vi "test_read-nmea-data2.vi"() -> ()   [LabVIEW 2019] (continued)
\t$GPGSV,3,2,09,09,45,074,34,12,24,277,32,17,33,153,39,19,53,157,39,1*6A\n\t\n15:11:33.42\tF9P\t$GPGSV,3,3,09,25,12,307,18,1*54\n\t\n15:11:33.44\tF9P\t$GPGSV,3,1,09,02,54,318,,04,18,044,,05,37,247,,06,64,047,22,6*6B\n\t\n15:11:33.46\tF9P\t$GPGSV,3,2,09,09,45,074,24,12,24,277,,17,33,153,23,19,53,157,,6*6C\n\t\n15:11:33.48\tF9P\t$GPGSV,3,3,09,25,12,307,,6*5A\n\t\n15:11:33.50\tF9P\t$GLGSV,2,1,08,69,12,031,,70,71,039,,71,52,205,32,72,04,209,,1*7B\n\t\n15:11:33.52\tF9P\t$GLGSV,2,2,08,77,01,326,,84,20,122,13,85,70,065,34,86,36,330,,1*7E\n\t\n15:11:33.54\tF9P\t$GLGSV,2,1,08,69,12,031,,70,71,039,,71,52,205,26,72,04,209,,3*7C\n\t\n15:11:33.56\tF9P\t$GLGSV,2,2,08,77,01,326,,84,20,122,17,85,70,065,23,86,36,330,,3*7E\n\t\n15:11:33.58\tF9P\t$GAGSV,2,1,08,02,08,297,08,04,66,118,32,09,32,193,25,11,71,358,20,7*75\n\t\n15:11:33.60\tF9P\t$GAGSV,2,2,08,12,40,102,32,19,26,045,19,25,09,249,,36,26,308,23,7*71\n\t\n15:11:33.62\tF9P\t$GAGSV,2,1,08,02,08,297,,04,66,118,,09,32,193,,11,71,358,,2*7C\n\t\n15:11:33.64\tF9P\t$GAGSV,2,2,08,12,40,102,,19,26,045,,25,09,249,,36,26,308,,2*7C\n\t\n15:11:33.66\tF9P\t$GBGSV,1,1,03,11,50,132,33,14,87,127,26,33,60,219,25,1*41\n\t\n15:11:33.68\tF9P\t$GBGSV,1,1,03,11,50,132,26,14,87,127,,33,60,219,,3*44\n\t\n15:11:33.70\tF9P\t$GNGLL,3723.52856,N,12656.91091,E,061135.00,A,A*78\n\t\n15:11:33.72\tF9P\t\t\n15:11:33.74\tF9P\t\t\n15:11:33.76\tF9P\t\t\n15:11:33.78\tF9P\t\t\n15:11:33.80\tF9P\t\t\n15:11:33.84\tF9P\t\t\n15:11:33.86\tF9P\t\t\n15:11:33.88\tF9P\t\t\n15:11:33.90\tF9P\t\t\n15:11:33.92\tF9P\t\t\n15:11:33.94\tF9P\t\t\n15:11:33.96\tF9P\t\t\n15:11:33.98\tF9P\t\t\n15:11:34.00\tF9P\t\t\n15:11:34.02\tF9P\t\t\n15:11:34.04\tF9P\t\t\n15:11:34.06\tF9P\t\t\n15:11:34.08\tF9P\t\t\n15:11:34.10\tF9P\t\t\n15:11:34.12\tF9P\t\t\n15:11:34.14\tF9P\t\t\n15:11:34.16\tF9P\t\t\n15:11:34.18\tF9P\t\t\n15:11:34.20\tF9P\t\t\n15:11:34.22\tF9P\t\t\n15:11:34.24\tF9P\t$GNRMC,061136.00,A,3723.52804,N,12656.91189,E,2.935,120.29,250720,,,A,V*0E\n\t\n15:11:34.26\tF9P\t$GNVTG,120.29,T,,M,2.935,N,5.436,K,A*22\n\t\n15:11:34.28\tF9P\t$GNGGA,061136.00,3723.52804,N,12656.91189,E,1,12,0.68,33.7,M,18.5,M,,*77\n\t\n15:11:34.30\tF9P\t$GNGSA,A,3,12,06,19,05,17,09,04,02,,,,,1.27,0.68,1.08,1*03\n\t\n15:11:34.32\tF9P\t$GNGSA,A,3,85,71,84,,,,,,,,,,1.27,0.68,1.08,2*06\n\t\n15:11:34.34\tF9P\t$GNGSA,A,3,36,19,11,04,09,12,,,,,,,1.27,0.68,1.08,3*03\n\t\n15:11:34.36\tF9P\t$GNGSA,A,3,14,11,33,,,,,,,,,,1.27,0.68,1.08,4*02\n\t\n15:11:34.38\tF9P\t$GPGSV,3,1,09,02,54,318,27,04,18,044,29,05,37,247,21,06,64,047,25,1*66\n\t\n15:11:34.40\tF9P\t$GPGSV,3,2,09,09,45,074,38,12,24,277,31,17,33,153,37,19,53,157,33,1*61\n\t\n15:11:34.42\tF9P\t$GPGSV,3,3,09,25,12,307,17,1*5B\n\t\n15:11:34.44\tF9P\t$GPGSV,3,1,09,02,54,318,,04,18,044,27,05,37,247,,06,64,047,21,6*6D\n\t\n15:11:34.46\tF9P\t$GPGSV,3,2,09,09,45,074,23,12,24,277,,17,33,153,23,19,53,157,,6*6B\n\t\n15:11:34.48\tF9P\t$GPGSV,3,3,09,25,12,307,,6*5A\n\t\n15:11:34.50\tF9P\t$GLGSV,2,1,08,69,12,031,,70,71,039,,71,52,205,28,72,04,209,,1*70\n\t\n15:11:34.52\tF9P\t$GLGSV,2,2,08,77,01,326,,84,20,122,10,85,70,065,35,86,36,330,,1*7C\n\t\n15:11:34.54\tF9P\t$GLGSV,2,1,08,69,12,031,,70,71,039,,71,52,205,23,72,04,209,,3*79\n\t\n15:11:34.56\tF9P\t$GLGSV,2,2,08,77,01,326,,84,20,122,18,85,70,065,23,86,36,330,,3*71\n\t\n15:11:34.58\tF9P\t$GAGSV,2,1,08,02,08,297,10,04,66,118,36,09,32,193,34,11,71,358,30,7*79\n\t\n15:11:34.60\tF9P\t$GAGSV,2,2,08,12,40,102,28,19,26,045,10,25,09,249,,36,26,308,24,7*74\n\t\n15:11:34.62\tF9P\t$GAGSV,2,1,08,02,08,297,,04,66,118,,09,32,193,,11,71,358,,2*7C\n\t\n15:11:34.64\tF9P\t$GAGSV,2,2,08,12,40,102,,19,26,045,,25,09,249,,36,26,308,,2*7C\n\t\n15:11:34.66\tF9P\t$GBGSV,1,1,03,11,50,132,33,14,87,127,26,33,60,219,30,1*45\n\t\n15:11:34.68\tF9P\t$GBGSV,1,1,03,11,50,132,,14,87,127,,33,60,219,,3*40\n\t\n15:11:34.70\tF9P\t$GNGLL,3723.52804,N,12656.91189,E,061136.00,A,A*74\n\t\n15:11:34.72\tF9P\t\t\n15:11:34.74\tF9P\t\t\n15:11:34.76\tF9P\t\t\n15:11:34.78\tF9P\t\t\n15:11:34.80\tF9P\t\t\n15:11:34.82\tF9P\t\t\n15:11:34.84\tF9P\t\t\n15:11:34.86\tF9P\t\t\n15:11:34.88\tF9P\t\t\n15:11:34.90\tF9P\t\t\n15:11:34.92\tF9P\t\t\n15:11:34.94\tF9P\t\t\n15:11:34.96\tF9P\t\t\n15:11:34.98\tF9P\t\t\n15:11:35.00\tF9P\t\t\n15:11:35.02\tF9P\t\t\n15:11:35.04\tF9P\t\t\n15:11:35.06\tF9P\t\t\n15:11:35.08\tF9P\t\t\n15:11:35.10\tF9P\t\t\n15:11:35.12\tF9P\t\t\n15:11:35.14\tF9P\t\t\n15:11:35.16\tF9P\t\t\n15:11:35.18\tF9P\t\t\n15:11:35.20\tF9P\t\t\n15:11:35.22\tF9P\t\t\n15:11:35.24\tF9P\t$GNRMC,061137.00,A,3723.52782,N,12656.91238,E,0.844,114.96,250720,,,A,V*01\n\t\n15:11:35.26\tF9P\t$GNVTG,114.96,T,,M,0.844,N,1.564,K,A*26\n\t\n15:11:35.28\tF9P\t$GNGGA,061137.00,3723.52782,N,12656.91238,E,1,12,0.68,33.5,M,18.5,M,,*7C\n\t\n15:11:35.30\tF9P\t$GNGSA,A,3,12,06,19,05,17,09,04,02,,,,,1.27,0.68,1.08,1*03\n\t\n15:11:35.32\tF9P\t$GNGSA,A,3,85,71,84,,,,,,,,,,1.27,0.68,1.08,2*06\n\t\n15:11:35.34\tF9P\t$GNGSA,A,3,36,19,11,04,09,12,,,,,,,1.27,0.68,1.08,3*03\n\t\n15:11:35.36\tF9P\t$GNGSA,A,3,14,11,33,,,,,,,,,,1.27,0.68,1.08,4*02\n\t\n15:11:35.38\tF9P\t$GPGSV,3,1,09,02,54,318,28,04,18,044,28,05,37,247,24,06,64,047,36,1*6F\n\t\n15:11:35.40\tF9P\t$GPGSV,3,2,09,09,45,074,42,12,24,277,31,17,33,153,40,19,53,157,27,1*69\n\t\n15:11:35.42\tF9P\t$GPGSV,3,3,09,25,12,307,16,1*5A\n\t\n15:11:35.44\tF9P\t$GPGSV,3,1,09,02,54,318,,04,18,044,25,05,37,247,,06,64,047,22,6*6C\n\t\n15:11:35.46\tF9P\t$GPGSV,3,2,09,09,45,074,29,12,24,277,,17,33,153,22,19,53,157,,6*60\n\t\n15:11:35.48\tF9P\t$GPGSV,3,3,09,25,12,307,,6*5A\n\t\n15:11:35.50\tF9P\t$GLGSV,2,1,08,69,12,031,,70,71,039,,71,52,205,21,72,04,209,,1*79\n\t\n15:11:35.52\tF9P\t$GLGSV,2,2,08,77,01,326,,84,20,122,14,85,70,065,32,86,36,330,,1*7F\n\t\n15:11:35.54\tF9P\t$GLGSV,2,1,08,69,12,031,,70,71,039,,71,52,205,22,72,04,209,,3*78\n\t\n15:11:35.56\tF9P\t$GLGSV,2,2,08,77,01,326,,84,20,122,18,85,70,065,23,86,36,330,,3*71\n\t\n15:11:35.58\tF9P\t$GAGSV,2,1,08,02,08,297,09,04,66,118,34,09,32,193,30,11,71,358,24,7*72\n\t\n15:11:35.60\tF9P\t$GAGSV,2,2,08,12,40,102,30,19,26,045,19,25,09,249,,36,26,308,29,7*79\n\t\n15:11:35.62\tF9P\t$GAGSV,2,1,08,02,08,297,,04,66,118,,09,32,193,,11,71,358,,2*7C\n\t\n15:11:35.64\tF9P\t$GAGSV,2,2,08,12,40,102,,19,26,045,,25,09,249,,36,26,308,,2*7C\n\t\n15:11:35.66\tF9P\t$GBGSV,1,1,03,11,50,132,36,14,87,127,31,33,60,219,29,1*4E\n\t\n15:11:35.68\tF9P\t$GBGSV,1,1,03,11,50,132,,14,87,127,,33,60,219,,3*40\n\t\n15:11:35.70\tF9P\t$GNGLL,3723.52782,N,12656.91238,E,061137.00,A,A*7D\n\t\n15:11:35.72\tF9P\t\t\n15:11:35.74\tF9P\t\t\n15:11:35.76\tF9P\t\t\n15:11:35.78\tF9P\t\t\n15:11:35.80\tF9P\t\t\n15:11:35.82\tF9P\t\t\n15:11:35.84\tF9P\t\t\n15:11:35.86\tF9P\t\t\n15:11:35.88\tF9P\t\t\n15:11:35.90\tF9P\t\t\n15:11:35.92\tF9P\t\t\n15:11:35.94\tF9P\t\t\n15:11:35.96\tF9P\t\t\n15:11:35.98\tF9P\t\t\n15:11:36.00\tF9P\t\t\n15:11:36.02\tF9P\t\t\n15:11:36.04\tF9P\t\t\n15:11:36.06\tF9P\t\t\n15:11:36.08\tF9P\t\t\n15:11:36.10\tF9P\t\t\n15:11:36.12\tF9P\t\t\n15:11:36.14\tF9P\t\t\n15:11:36.16\tF9P\t\t\n15:11:36.18\tF9P\t\t\n15:11:36.20\tF9P\t\t\n15:11:36.22\tF9P\t\t\n15:11:36.24\tF9P\t$GNRMC,061138.00,A,3723.52726,N,12656.91274,E,2.515,150.84,25072\t\n15:11:36.26\tF9P\t0,,,A,V*00\n\t\n15:11:36.28\tF9P\t$GNVTG,150.84,T,,M,2.515,N,4.658,K,A*27\n\t\n15:11:36.30\tF9P\t$GNGGA,061138.00,3723.52726,N,12656.91274,E,1,12,0.71,34.0,M,18.5,M,,*7F\n\t\n15:11:36.32\tF9P\t$GNGSA,A,3,12,06,19,05,17,09,04,02,,,,,1.29,0.71,1.08,1*05\n\t\n15:11:36.34\tF9P\t$GNGSA,A,3,85,71,84,,,,,,,,,,1.29,0.71,1.08,2*00\n\t\n15:11:36.36\tF9P\t$GNGSA,A,3,36,19,11,04,09,12,,,,,,,1.29,0.71,1.08,3*05\n\t\n15:11:36.38\tF9P\t$GNGSA,A,3,14,11,33,,,,,,,,,,1.29,0.71,1.08,4*04\n\t\n15:11:36.40\tF9P\t$GPGSV,3,1,09,02,54,318,33,04,18,044,29,05,37,247,24,06,64,047,40,1*65\n\t\n15:11:36.43\tF9P\t$GPGSV,3,2,09,09,45,074,38,12,24,277,28,17,33,153,42,19,53,157,32,1*6A\n\t\n15:11:36.45\tF9P\t$GPGSV,3,3,09,25,12,307,15,1*59\n\t\n15:11:36.47\tF9P\t$GPGSV,3,1,09,02,54,318,,04,18,044,21,05,37,247,,06,64,047,22,6*68\n\t\n15:11:36.49\tF9P\t$GPGSV,3,2,09,09,45,074,26,12,24,277,22,17,33,153,29,19,53,157,,6*64\n\t\n15:11:36.51\tF9P\t$GPGSV,3,3,09,25,12,307,,6*5A\n\t\n15:11:36.53\tF9P\t$GLGSV,2,1,08,69,12,031,,70,71,039,,71,52,205,29,72,04,209,,1*71\n\t\n15:11:36.55\tF9P\t$GLGSV,2,2,08,77,01,326,,84,20,122,07,85,70,065,38,86,36,330,,1*77\n\t\n15:11:36.57\tF9P\t$GLGSV,2,1,08,69,12,031,,70,71,039,,71,52,205,25,72,04,209,,3*7F\n\t\n15:11:36.59\tF9P\t$GLGSV,2,2,08,77,01,326,,84,20,122,18,85,70,065,24,86,36,330,,3*76\n\t\n15:11:36.61\tF9P\t$GAGSV,2,1,08,02,08,297,10,04,66,118,21,09,32,193,25,11,71,358,24,7*7A\n\t\n15:11:36.63\tF9P\t$GAGSV,2,2,08,12,40,102,29,19,26,045,18,25,09,249,,36,26,308,19,7*73\n\t\n15:11:36.65\tF9P\t$GAGSV,2,1,08,02,08,297,,04,66,118,,09,32,193,,11,71,358,,2*7C\n\t\n15:11:36.67\tF9P\t$GAGSV,2,2,08,12,40,102,,19,26,045,,25,09,249,,36,26,308,,2*7C\n\t\n15:11:36.69\tF9P\t$GBGSV,1,1,03,11,50,132,33,14,87,127,30,33,60,219,28,1*4B\n\t\n15:11:36.71\tF9P\t$GBGSV,1,1,03,11,50,132,36,14,87,127,,33,60,219,,3*45\n\t\n15:11:36.73\tF9P\t$GNGLL,3723.52726,N,12656.91274,E,061138.00,A,A*74\n\t\n15:11:36.75\tF9P\t\t\n15:11:36.77\tF9P\t\t\n15:11:36.79\tF9P\t\t\n15:11:36.81\tF9P\t\t\n15:11:36.83\tF9P\t\t\n15:11:36.85\tF9P\t\t\n15:11:36.87\tF9P\t\t\n15:11:36.89\tF9P\t\t\n15:11:36.91\tF9P\t\t\n15:11:36.93\tF9P\t\t\n15:11:36.95\tF9P\t\t\n15:11:36.97\tF9P\t\t\n15:11:36.99\tF9P\t\t\n15:11:37.01\tF9P\t\t\n15:11:37.03\tF9P\t\t\n15:11:37.05\tF9P\t\t\n15:11:37.07\tF9P\t\t\n15:11:37.09\tF9P\t\t\n15:11:37.11\tF9P\t\t\n15:11:37.13\tF9P\t\t\n15:11:37.15\tF9P\t\t\n15:11:37.17\tF9P\t\t\n15:11:37.19\tF9P\t\t\n15:11:37.21\tF9P\t\t\n15:11:37.23\tF9P\t\t\n15:11:37.25\tF9P\t$GNRMC,061139.00,A,3723.52691,N,12656.91315,E,0.968,139.94,250720,,,A,V*00\n\t\n15:11:37.27\tF9P\t$GNVTG,139.94,T,,M,0.968,N,1.792,K,A*2F\n\t\n15:11:37.29\tF9P\t$GNGGA,061139.00,3723.52691,N,12656.91315,E,1,12,0.71,34.1,M,18.5,M,,*74\n\t\n15:11:37.31\tF9P\t$GNGSA,A,3,12,06,19,05,17,09,04,02,,,,,1.29,0.71,1.08,1*05\n\t\n15:11:37.33\tF9P\t$GNGSA,A,3,85,71,84,,,,,,,,,,1.29,0.71,1.08,2*00\n\t\n15:11:37.35\tF9P\t$GNGSA,A,3,36,19,11,04,09,12,,,,,,,1.29,0.71,1.08,3*05\n\t\n15:11:37.37\tF9P\t$GNGSA,A,3,14,11,33,,,,,,,,,,1.29,0.71,1.08,4*04\n\t\n15:11:37.39\tF9P\t$GPGSV,3,1,09,02,54,318,29,04,18,044,22,05,37,247,23,06,64,047,38,1*6D\n\t\n15:11:37.41\tF9P\t$GPGSV,3,2,09,09,45,074,39,12,24,277,27,17,33,153,39,19,53,157,27,1*6C\n\t\n15:11:37.43\tF9P\t$GPGSV,3,3,09,25,12,307,15,1*59\n\t\n15:11:37.45\tF9P\t$GPGSV,3,1,09,02,54,318,,04,18,044,19,05,37,247,,06,64,047,21,6*60\n\t\n15:11:37.47\tF9P\t$GPGSV,3,2,09,09,45,074,26,12,24,277,20,17,33,153,29,19,53,157,,6*66\n\t\n15:11:37.49\tF9P\t$GPGSV,3,3,09,25,12,307,,6*5A\n\t\n15:11:37.51\tF9P\t$GLGSV,2,1,08,69,12,031,,70,71,039,,71,52,205,29,72,04,209,,1*71\n\t\n15:11:37.53\tF9P\t$GLGSV,2,2,08,77,01,326,,84,20,122,10,85,70,065,34,86,36,330,,1*7D\n\t\n15:11:37.55\tF9P\t$GLGSV,2,1,08,69,12,031,,70,71,039,,71,52,205,23,72,04,209,,3*79\n\t\n15:11:37.57\tF9P\t$GLGSV,2,2,08,77,01,326,,84,20,122,18,85,70,065,22,86,36,330,,3*70\n\t\n15:11:37.59\tF9P\t$GAGSV,2,1,08,02,08,297,10,04,66,118,30,09,32,193,26,11,71,358,24,7*79\n\t\n15:11:37.61\tF9P\t$GAGSV,2,2,08,12,40,102,23,19,26,045,19,25,09,249,,36,26,308,21,7*73\n\t\n15:11:37.63\tF9P\t$GAGSV,2,1,08,02,08,297,,04,66,118,28,09,32,193,,11,71,358,,2*76\n\t\n15:11:37.65\tF9P\t$GAGSV,2,2,08,12,40,102,,19,26,045,,25,09,249,,36,26,308,,2*7C\n\t\n15:11:37.67\tF9P\t$GBGSV,1,1,03,11,50,132,29,14,87,127,24,33,60,219,28,1*45\n\t\n15:11:37.69\tF9P\t$GBGSV,1,1,03,11,50,132,36,14,87,127,,33,60,219,,3*45\n\t\n15:11:37.71\tF9P\t$GNGLL,3723.52691,N,12656.91315,E,061139.00,A,A*7E\n\t\n15:11:37.73\tF9P\t\t\n15:11:37.75\tF9P\t\t\n15:11:37.77\tF9P\t\t\n15:11:37.79\tF9P\t\t\n15:11:37.81\tF9P\t\t\n15:11:37.83\tF9P\t\t\n15:11:37.85\tF9P\t\t\n15:11:37.87\tF9P\t\t\n15:11:37.89\tF9P\t\t\n15:11:37.91\tF9P\t\t\n15:11:37.93\tF9P\t\t\n15:11:37.95\tF9P\t\t\n15:11:37.97\tF9P\t\t\n15:11:37.99\tF9P\t\t\n15:11:38.01\tF9P\t\t\n15:11:38.03\tF9P\t\t\n15:11:38.05\tF9P\t\t\n15:11:38.07\tF9P\t\t\n15:11:38.09\tF9P\t\t\n15:11:38.11\tF9P\t\t\n15:11:38.13\tF9P\t\t\n15:11:38.15\tF9P\t\t\n15:11:38.17\tF9P\t\t\n15:11:38.19\tF9P\t\t\n15:11:38.21\tF9P\t\t\n15:11:38.23\tF9P\t\t\n15:11:38.25\tF9P\t$GNRMC,061140.00,A,3723.52674,N,12656.91342,E,0.860,,250720,,,A,V*16\n\t\n15:11:38.27\tF9P\t$GNVTG,,T,,M,0.860,N,1.593,K,A*3D\n\t\n15:11:38.29\tF9P\t$GNGGA,061140.00,3723.52674,N,12656.91342,E,1,12,0.74,34.5,M,18.5,M,,*72\n\t\n15:11:38.31\tF9P\t$GNGSA,A,3,12,06,19,05,17,09,04,02,,,,,1.44,0.74,1.23,1*02\n\t\n15:11:38.33\tF9P\t$GNGSA,A,3,85,71,84,,,,,,,,,,1.44,0.74,1.23,2*07\n\t\n15:11:38.35\tF9P\t$GNGSA,A,3,36,19,11,04,09,12,,,,,,,1.44,0.74,1.23,3*02\n\t\n15:11:38.37\tF9P\t$GNGSA,A,3,14,11,33,,,,,,,,,,1.44,0.74,1.23,4*03\n\t\n15:11:38.39\tF9P\t$GPGSV,3,1,09,02,54,318,30,04,18,044,23,05,37,247,21,06,64,047,41,1*68\n\t\n15:11:38.41\tF9P\t$GPGSV,3,2,09,09,45,074,36,12,24,277,26,17,33,153,32,19,53,157,30,1*6F\n\t\n15:11:38.43\tF9P\t$GPGSV,3,3,09,25,12,307,17,1*5B\n\t\n15:11:38.45\tF9P\t$GPGSV,3,1,09,02,54,318,,04,18,044,17,05,37,247,,06,64,047,22,6*6D\n\t\n15:11:38.47\tF9P\t$GPGSV,3,2,09,09,45,074,26,12,24,277,20,17,33,153,29,19,53,157,,6*66\n\t\n15:11:38.49\tF9P\t$GPGSV,3,3,09,25,12,307,,6*5A\n\t\n15:11:38.51\tF9P\t$GLGSV,2,1,08,69,12,031,,70,71,039,,71,52,205,28,72,04,209,,1*70\n\t\n15:11:38.53\tF9P\t$GLGSV,2,2,08,77,01,326,,84,20,122,10,85,70,065,31,86,36,330,,1*78\n\t\n15:11:38.55\tF9P\t$GLGSV,2,1,08,69,12,031,,70,71,039,,71,52,205,22,72,04,209,,3*78\n\t\n15:11:38.57\tF9P\t$GLGSV,2,2,08,77,01,326,,84,20,122,18,85,70,065,22,86,36,330,,3*70\n\t\n15:11:38.59\tF9P\t$GAGSV,2,1,08,02,08,297,06,04,66,118,25,09,32,193,25,11,71,358,24,7*79\n\t\n15:11:38.61\tF9P\t$GAGSV,2,2,08,12,40,102,25,19,26,045,22,25,09,249,,36,26,308,22,7*7E\n\t\n15:11:38.63\tF9P\t$GAGSV,2,1,08,02,08,297,,04,66,118,27,09,32,193,,11,71,358,,2*79\n\t\n15:11:38.65\tF9P\t$GAGSV,2,2,08,12,40,102,,19,26,045,,25,09,249,,36,26,308,,2*7C\n\t\n15:11:38.67\tF9P\t$GBGSV,1,1,03,11,50,132,36,14,87,127,25,33,60,219,26,1*44\n\t\n15:11:38.69\tF9P\t$GBGSV,1,1,03,11,50,132,33,14,87,127,,33,60,219,,3*40\n\t\n15:11:38.71\tF9P\t$GNGLL,3723.52674,N,12656.91342,E,061140.00,A,A*79\n\t\n15:11:38.73\tF9P\t\t\n15:11:38.75\tF9P\t\t\n15:11:38.77\tF9P\t\t\n15:11:38.79\tF9P\t\t\n15:11:38.81\tF9P\t\t\n15:11:38.83\tF9P\t\t\n15:11:38.85\tF9P\t\t\n15:11:38.87\tF9P\t\t\n15:11:38.89\tF9P\t\t\n15:11:38.91\tF9P\t\t\n15:11:38.93\tF9P\t\t\n15:11:38.95\tF9P\t\t\n15:11:38.97\tF9P\t\t\n15:11:38.99\tF9P\t\t\n15:11:39.01\tF9P\t\t\n15:11:39.03\tF9P\t\t\n15:11:39.05\tF9P\t\t\n15:11:39.07\tF9P\t\t\n15:11:39.09\tF9P\t\t\n15:11:39.11\tF9P\t\t\n15:11:39.13\tF9P\t\t\n15:11:39.15\tF9P\t\t\n15:11:39.17\tF9P\t\t\n15:11:39.19\tF9P\t\t\n15:11:39.21\tF9P\t\t\n15:11:39.23\tF9P\t\t\n15:11:39.25\tF9P\t$GNRMC,061141.00,A,3723.52639,N,12656.91381,E,1.583,133.93,250720,,,A,V*05\n\t\n15:11:39.27\tF9P\t$GNVTG,133.93,T,,M,1.583,N,2.932,K,A*2D\n\t\n15:11:39.29\tF9P\t$GNGGA,061141.00,3723.52639,N,12656.91381,E,1,12,0.71,35.1,M,18.5,M,,*75\n\t\n15:11:39.31\tF9P\t$GNGSA,A,3,12,06,19,05,17,09,04,02,,,,,1.29,0.71,1.08,1*05\n\t\n15:11:39.33\tF9P\t$GNGSA,A,3,85,71,84,,,,,,,,,,1.29,0.71,1.08,2*00\n\t\n15:11:39.35\tF9P\t$GNGSA,A,3,36,19,11,04,09,12,,,,,,,1.29,0.71,1.08,3*05\n\t\n15:11:39.37\tF9P\t$GNGSA,A,3,14,11,33,,,,,,,,,,1.29,0.71,1.08,4*04\n\t\n15:11:39.39\tF9P\t$GPGSV,3,1,09,02,54,318,31,04,18,044,23,05,37,247,22,06,64,047,32,1*6E\n\t\n15:11:39.41\tF9P\t$GPGSV,3,2,09,09,45,074,35,12,24,277,40,17,33,153,32,19,53,157,30,1*6C\n\t\n15:11:39.43\tF9P\t$GPGSV,3,3,09,25,12,307,18,1*54\n\t\n15:11:39.45\tF9P\t$GPGSV,3,1,09,02,54,318,,04,18,044,17,05,37,247,,06,64,047,23,6*6C\n\t\n15:11:39.47\tF9P\t$GPGSV,3,2,09,09,45,074,32,12,24,277,22,17,33,153,20,19,53,157,,6*68\n\t\n15:11:39.49\tF9P\t$GPGSV,3,3,09,25,12,307,,6*5A\n\t\n15:11:39.51\tF9P\t$GLGSV,2,1,08,69,12,031,,70,71,039,,71,52,205,33,72,04,209,,1*7A\n\t\n15:11:39.53\tF9P\t$GLGSV,2,2,08,77,01,326,,84,20,122,09,85,70,065,28,86,36,330,,1*78\n\t\n15:11:39.55\tF9P\t$GLGSV,2,1,08,69,12,031,,70,71,039,,71,52,205,22,72,04,209,,3*78\n\t\n15:11:39.57\tF9P\t$GLGSV,2,2,08,77,01,326,,84,20,122,17,85,70,065,20,86,36,330,,3*7D\n\t\n15:11:39.59\tF9P\t$GAGSV,2,1,08,02,08,297,10,04,66,118,29,09,32,193,28,11,71,358,25,7*7E\n\t\n15:11:39.61\tF9P\t$GAGSV,2,2,08,12,40,102,26,19,26,045,22,25,09,249,,36,26,308,36,7*78\n\t\n15:11:39.63\tF9P\t$GAGSV,2,1,08,02,08,297,,04,66,118,28,09,32,193,,11,71,358,,2*76\n\t\n15:11:39.65\tF9P\t$GAGSV,2,2,08,12,40,102,,19,26,045,,25,09,249,,36,26,308,,2*7C\n\t\n15:11:39.67\tF9P\t$GBGSV,1,1,03,11,50,132,32,14,87,127,25,33,60,219,27,1*41\n\t\n15:11:39.69\tF9P\t$GBGSV,1,1,03,11,50,132,28,14,87,127,,33,60,219,,3*4A\n\t\n15:11:39.71\tF9P\t$GNGLL,3723.52639,N,12656.91381,E,061141.00,A,A*7E\n\t\n15:11:39.73\tF9P\t\t\n15:11:39.75\tF9P\t\t\n15:11:39.77\tF9P\t\t\n15:11:39.79\tF9P\t\t\n15:11:39.81\tF9P\t\t\n15:11:39.83\tF9P\t\t\n15:11:39.85\tF9P\t\t\n15:11:39.87\tF9P\t\t\n15:11:39.89\tF9P\t\t\n15:11:39.91\tF9P\t\t\n15:11:39.93\tF9P\t\t\n15:11:39.95\tF9P\t\t\n15:11:39.97\tF9P\t\t\n15:11:39.99\tF9P\t\t\n15:11:40.01\tF9P\t\t\n15:11:40.03\tF9P\t\t\n15:11:40.05\tF9P\t\t\n15:11:40.07\tF9P\t\t\n15:11:40.09\tF9P\t\t\n15:11:40.11\tF9P\t\t\n15:11:40.13\tF9P\t\t\n15:11:40.15\tF9P\t\t\n15:11:40.17\tF9P\t\t\n15:11:40.19\tF9P\t\t\n15:11:40.21\tF9P\t\t\n15:11:40.23\tF9P\t\t\n15:11:40.25\tF9P\t$GNRMC,061142.00,A,3723.52609,N,12656.91430,E,1.915,119.31,250720,,,A,V*0B\n\t\n15:11:40.27\tF9P\t$GNVTG,119.31,T,,M,1.915,N,3.546,K,A*20\n\t\n15:11:40.29\tF9P\t$GNGGA,061142.00,3723.52609,N,12656.91430,E,1,12,0.71,34.9,M,18.5,M,,*71\n\t\n15:11:40.31\tF9P\t$GNGSA,A,3,12,06,19,05,17,09,04,02,,,,,1.29,0.71,1.08,1*05\n\t\n15:11:40.33\tF9P\t$GNGSA,A,3,85,71,84,,,,,,,,,,1.29,0.71,1.08,2*00\n\t\n15:11:40.35\tF9P\t$GNGSA,A,3,36,19,11,04,09,12,,,,,,,1.29,0.71,1.08,3*05\n\t\n15:11:40.37\tF9P\t$GNGSA,A,3,14,11,33,,,,,,,,,,1.29,0.71,1.08,4*04\n\t\n15:11:40.39\tF9P\t$GPGSV,3,1,09,02,54,318,38,04,18,044,22,05,37,247,22,06,64,047,32,1*66\n\t\n15:11:40.41\tF9P\t$GPGSV,3,2,09,09,45,074,34,12,24,277,37,17,33,153,33,19,53,157,26,1*6B\n\t\n15:11:40.43\tF9P\t$GPGSV,3,3,09,25,12,307,20,1*5F\n\t\n15:11:40.45\tF9P\t$GPGSV,3,1,09,02,54,318,,04,18,044,16,05,37,247,,06,64,047,22,6*6C\n\t\n15:11:40.47\tF9P\t$GPGSV,3,2,09,09,45,074,25,12,24,277,23,17,33,153,28,19,53,157,,6*67\n\t\n15:11:40.49\tF9P\t$GPGSV,3,3,09,25,12,307,,6*5A\n\t\n15:11:40.51\tF9P\t$GLGSV,2,1,08,69,12,031,,70,71,039,,71,52,205,32,72,04,209,,1*7B\n\t\n15:11:40.53\tF9P\t$GLGSV,2,2,08,77,01,326,,84,20,122,08,85,70,065,27,86,36,330,,1*76\n\t\n15:11:40.55\tF9P\t$GLGSV,2,1,08,69,12,031,,70,71,039,,71,52,205,23,72,04,209,,3*79\n\t\n15:11:40.57\tF9P\t$GLGSV,2,2,08,77,01,326,,84,20,122,17,85,70,065,21,86,36,330,,3*7C\n\t\n15:11:40.59\tF9P\t$GAGSV,2,1,08,02,08,297,09,04,66,118,29,09,32,193,28,11,71,358,26,7*75\n\t\n15:11:40.61\tF9P\t$GAGSV,2,2,08,12,40,102,27,19,26,045,22,25,09,249,,36,26,308,39,7*76\n\t\n15:11:40.63\tF9P\t$GAGSV,2,1,08,02,08,297,,04,66,118,31,09,32,193,,11,71,358,,2*7E\n\t\n15:11:40.65\tF9P\t$GAGSV,2,2,08,12,40,102,,19,26,045,,25,09,249,,36,26,308,,2*7C\n\t\n15:11:40.67\tF9P\t$GBGSV,1,1,03,11,50,132,28,14,87,127,26,33,60,219,32,1*4D\n\t\n15:11:40.69\tF9P\t$GBGSV,1,1,03,11,50,132,33,14,87,127,,33,60,219,,3*40\n\t\n15:11:40.71\tF9P\t$GNGLL,3723.52609,N,12656.91430,E,061142.00,A,A*73\n\t\n15:11:40.73\tF9P\t\t\n15:11:40.75\tF9P\t\t\n15:11:40.77\tF9P\t\t\n15:11:40.79\tF9P\t\t\n15:11:40.81\tF9P\t\t\n15:11:40.83\tF9P\t\t\n15:11:40.85\tF9P\t\t\n15:11:40.87\tF9P\t\t\n15:11:40.89\tF9P\t\t\n15:11:40.91\tF9P\t\t\n15:11:40.93\tF9P\t\t\n15:11:40.95\tF9P\t\t\n15:11:40.97\tF9P\t\t\n15:11:40.99\tF9P\t\t\n15:11:41.01\tF9P\t\t\n15:11:41.03\tF9P\t\t\n15:11:41.05\tF9P\t\t\n15:11:41.07\tF9P\t\t\n15:11:41.09\tF9P\t\t\n15:11:41.11\tF9P\t\t\n15:11:41.13\tF9P\t\t\n15:11:41.15\tF9P\t\t\n15:11:41.17\tF9P\t\t\n15:11:41.19\tF9P\t\t\n15:11:41.21\tF9P\t\t\n15:11:41.23\tF9P\t\t\n15:11:41.25\tF9P\t$GNRMC,061143.00,A,3723.52576,N,12656.91469,E,1.416,119.70,250720,,,A,V*06\n\t\n15:11:41.27\tF9P\t$GNVTG,119.70,T,,M,1.416,N,2.622,K,A*2B\n\t\n15:11:41.29\tF9P\t$GNGGA,061143.00,3723.52576,N,12656.91469,E,1,12,0.74,35.2,M,18.5,M,,*78\n
